vi "Periodic Tasks.vi"(8 "error in":errorcluster) -> ()   [LabVIEW 2020]
doc: "This VI runs in parallel to other tasks. It can contain as many user-defined periodic loops as you need. These can carry out PID or other sorts of timed response."
uses:
  <vilib>/Rock Robotics/WPI/ThirdParty/Phoenix-LabVIEW/Motor Controller/Controls/CTRE_Phoenix_MotorControl_ControlMode.ctl
  swerve_globals.vi
  shooter_globals.vi
  magazine_globals.vi
  climber_globals.vi
  <vilib>/Rock Robotics/WPI/ThirdParty/Phoenix-LabVIEW/Motor Controller/Get/CTRE_Phoenix_MotorController_GetSelectedSensorData.vi
  <vilib>/Rock Robotics/Network Tables/NT Write Number.vi
  <vilib>/Rock Robotics/Network Tables/NT Read Number.vi
  <vilib>/addons/control/pid/pid.llb/PID (DBL).vi
  <vilib>/Rock Robotics/WPI/Utilities/WPI_GetSetVariantRefNum.vi
  TitanLib/Lib/TitanLib.lvlib
  <vilib>/addons/control/pid/NI_PID_pid.lvlib
  <vilib>/Rock Robotics/WPI/ThirdParty/Phoenix-LabVIEW/Motor Controller/Get/CTRE_Phoenix_MotorController_GetVoltage.vi
panel:
  out "Theta":dbl
  in  "Enable Hood":bool
  out "Distance (in)":dbl
  out "Pressure Sensors":T1
  out "Analog  Sensors":cluster{"Analog 0 (V)":dbl, "Analog 1 (V)":dbl}
  in  "Start Compressor":bool
  in  "Stop Compressor":bool
  out "Position (Deg) 2":dbl format="%.2f"
  in  "Zero Turret Encoder 2":bool
  in  "Auto Turret 2":bool
  in  "Min Rotation (deg) 2":dbl=-25.0
  in  "Max Rotation (deg) 2":dbl=20.0
  in  "PID gains":T2={"proportional gain (Kc)"=0.05, "integral time (Ti, min)"=0.0, "derivative time (Td, min)"=0.0} {"derivative time (Td, min)" format="%.3g"; "integral time (Ti, min)" format="%.3e"; "proportional gain (Kc)" format="%.3g"}
  out "tx 2":dbl
  in  "Power Min":dbl
  in  "Climber Up Pos":dbl=-9.82
  in  "Climber Down Pos":dbl=-0.5
  in  "limelight constant":dbl=0.5
  out "Percent Output":dbl(graph)
  out "Setpoint (Deg)":dbl format="%.2f"
  in  "Constants":T3={"Set Constants"=FALSE, "P"=0.05, "I"=0.0, "D"=0.0, "F"=0.0, "I Zone"=0.0, "Cruise Velocity"=500000, "Acceleration"=500000, "Percent Deadband"=0.0}
  out "tx":dbl
  out "Position (Deg)":dbl format="%.2f"
  in  "Zero Turret Encoder":bool
  in  "Min Rotation (deg)":dbl=-45.0
  in  "Max Rotation (deg)":dbl=20.0
  in  "Auto Turret":bool
  out "Loop Time (ms)":u32(graph)
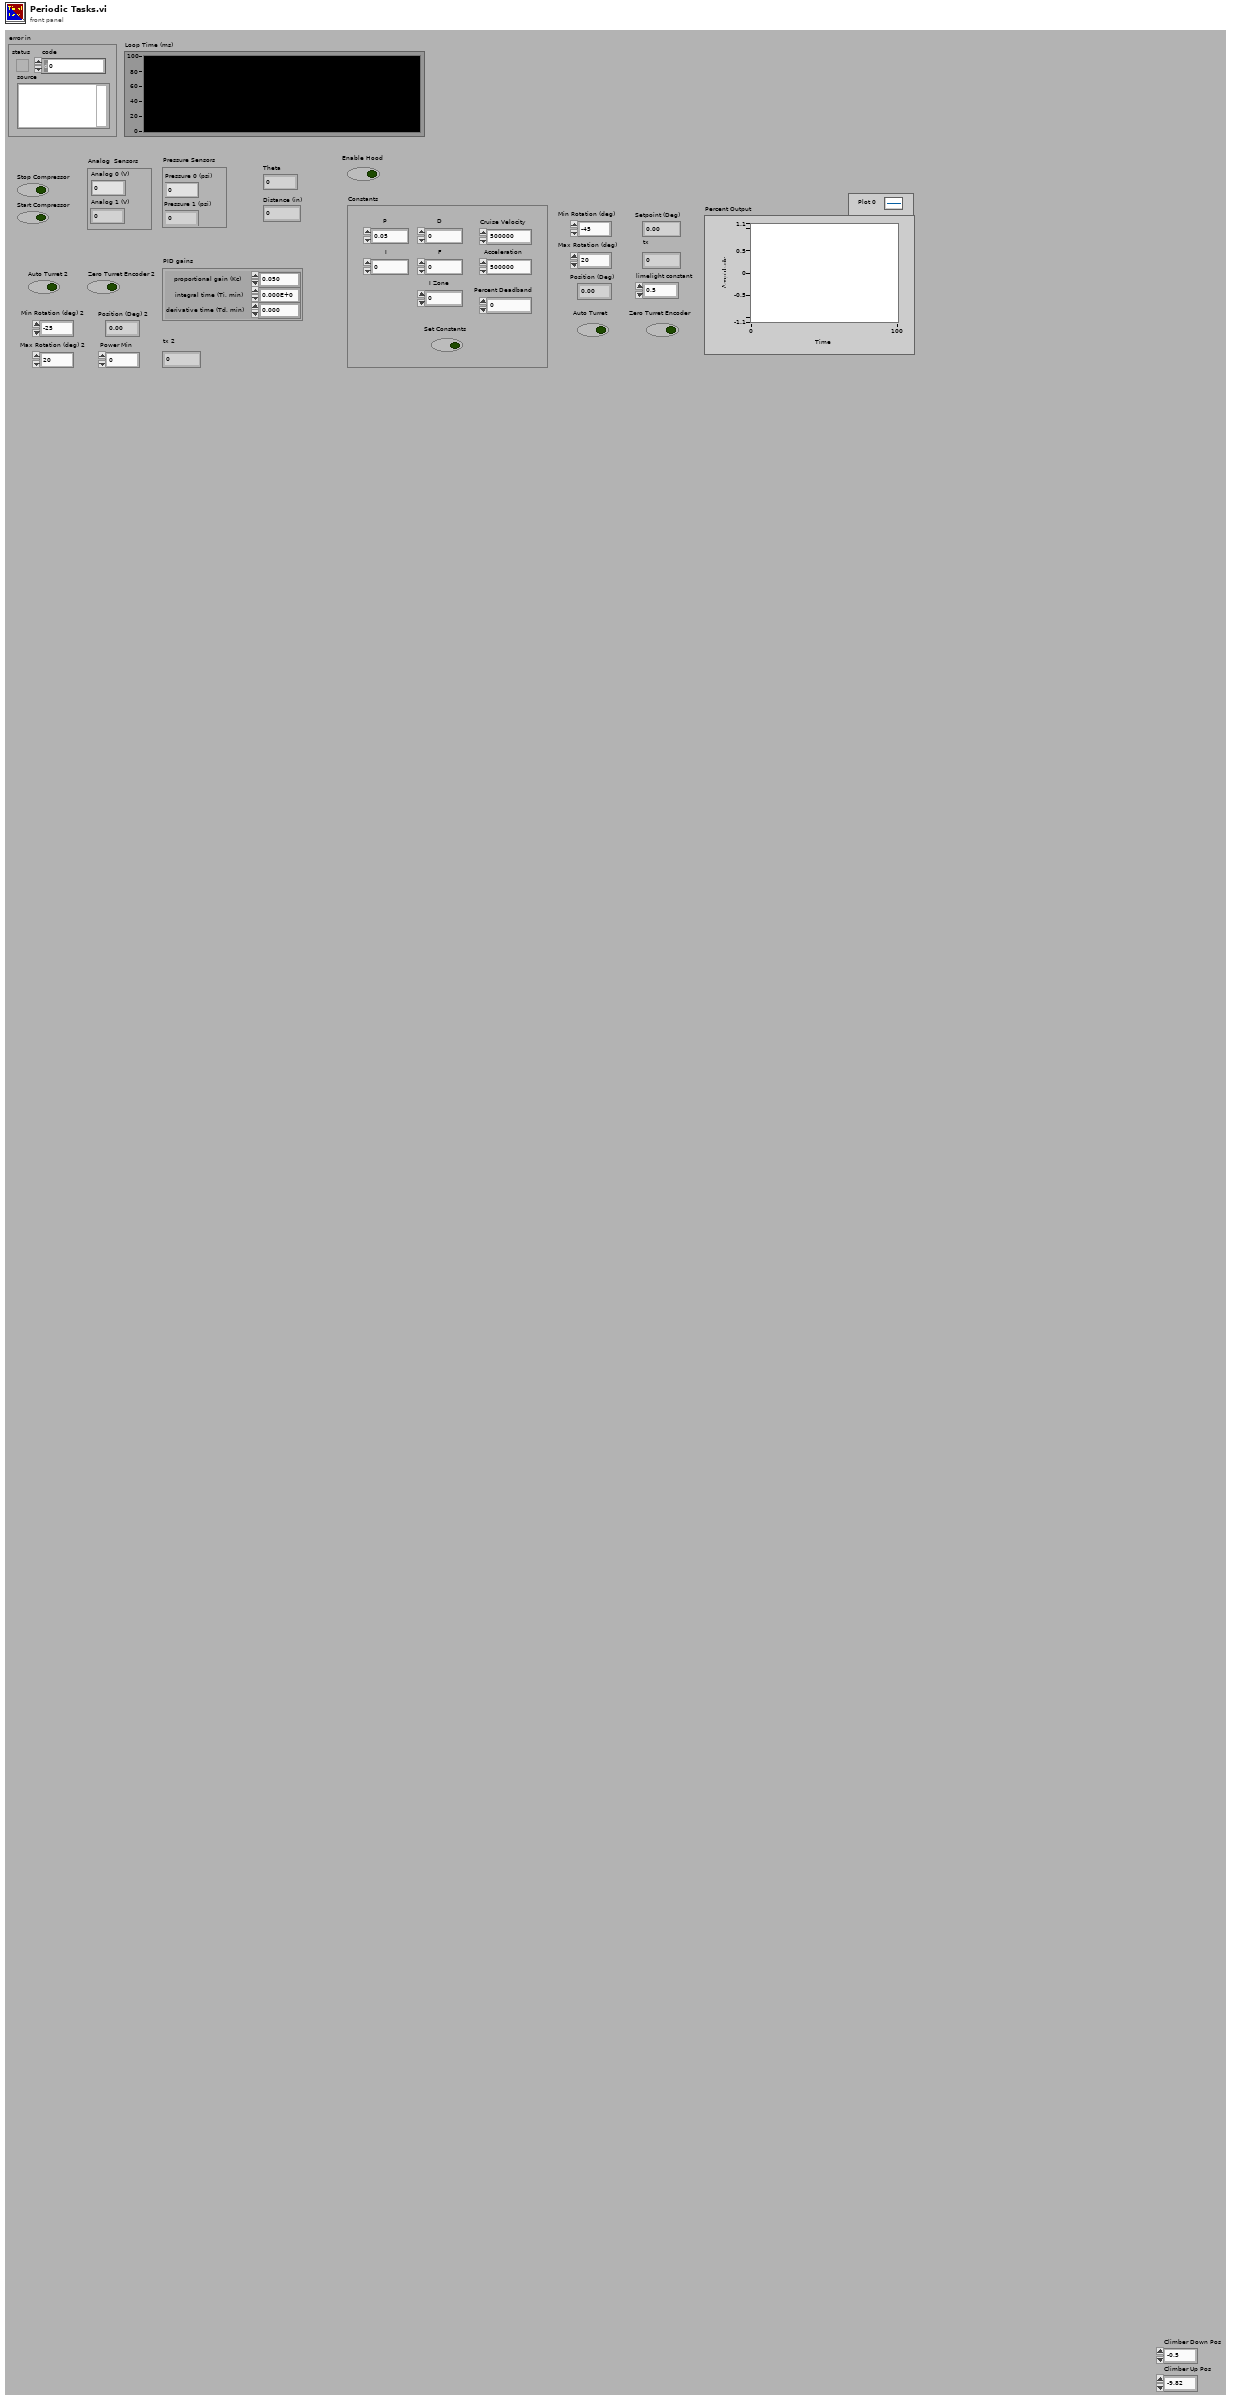
[diagram p1: front panel]
types:
  T1 = cluster{"Pressure 0 (psi)":dbl, "Pressure 1 (psi)":dbl}
  T2 = cluster{"proportional gain (Kc)":dbl, "integral time (Ti, min)":dbl, "derivative time (Td, min)":dbl}
  T3 = cluster{"Set Constants":bool, "P":dbl, "I":dbl, "D":dbl, "F":dbl, "I Zone":dbl, "Cruise Velocity":i32, "Acceleration":i32, "Percent Deadband":dbl}
  T4 = typedef "WPI_CompressorDevRef.ctl" = cluster{"DevStatus":errorcluster, "Pneumatics Control Module":u8}
  T5 = typedef "WPI_MotorControlDeviceRef.ctl" = cluster{"DeviceStatus":errorcluster, "Type":T6, "PWM":cluster{"PWM Channel":T7, "DeadBand":T8}, "CAN":cluster{"Device Number":u8, "SetOutput VI Ref":variant, "GetOutput VI Ref":variant, "Enable VI Ref":variant, "Disable VI Ref":variant, "Data":variant}, "Invert":bool, "DIO PWM":cluster{"PWM \"Enable\" Channel":T7, "DIOChannel":T9, "PWM Rate":dbl}}
  T6 = typedef "WPI_MotorControlType.ctl" = enum16{"PWM", "CAN", "DIO PWM"}
  T7 = typedef "FPGA_DIOPWMChannel.ctl" = enum8{"PWM 0", "PWM 1", "PWM 2", "PWM 3", "PWM 4", "PWM 5", "PWM 6", "PWM 7", "PWM 8", "PWM 9", "PWM MXP 0", "PWM MXP 1", "PWM MXP 2", "PWM MXP 3", "PWM MXP 4", "PWM MXP 5", "PWM MXP 6", "PWM MXP 7", "PWM MXP 8", "PWM MXP 9", "Invalid"}
  T8 = typedef "WPI_PWMDeadband.ctl" = cluster{"Name":string, "maxPositivePwm":i32, "minPositivePwm":i32, "centerPwm":i32, "maxNegativePwm":i32, "minNegativePwm":i32, "angularRange":u16}
  T9 = typedef "FPGA_DIOChannel.ctl" = enum8{"DIO 0", "DIO 1", "DIO 2", "DIO 3", "DIO 4", "DIO 5", "DIO 6", "DIO 7", "DIO 8", "DIO 9", "DIO MXP 0", "DIO MXP 1", "DIO MXP 2", "DIO MXP 3", "DIO MXP 4", "DIO MXP 5", "DIO MXP 6", "DIO MXP 7", "DIO MXP 8", "DIO MXP 9", "DIO MXP 10", "DIO MXP 11", "DIO MXP 12", "DIO MXP 13", "DIO MXP 14", "DIO MXP 15", "SPI Port CS1", "SPI Port CS2", "SPI Port CS3", "SPI Port MISO", "SPI Port MOSI", "Invalid"}
  T10 = typedef "CTRE_Phoenix_MotorControl_ControlMode.ctl" = u16
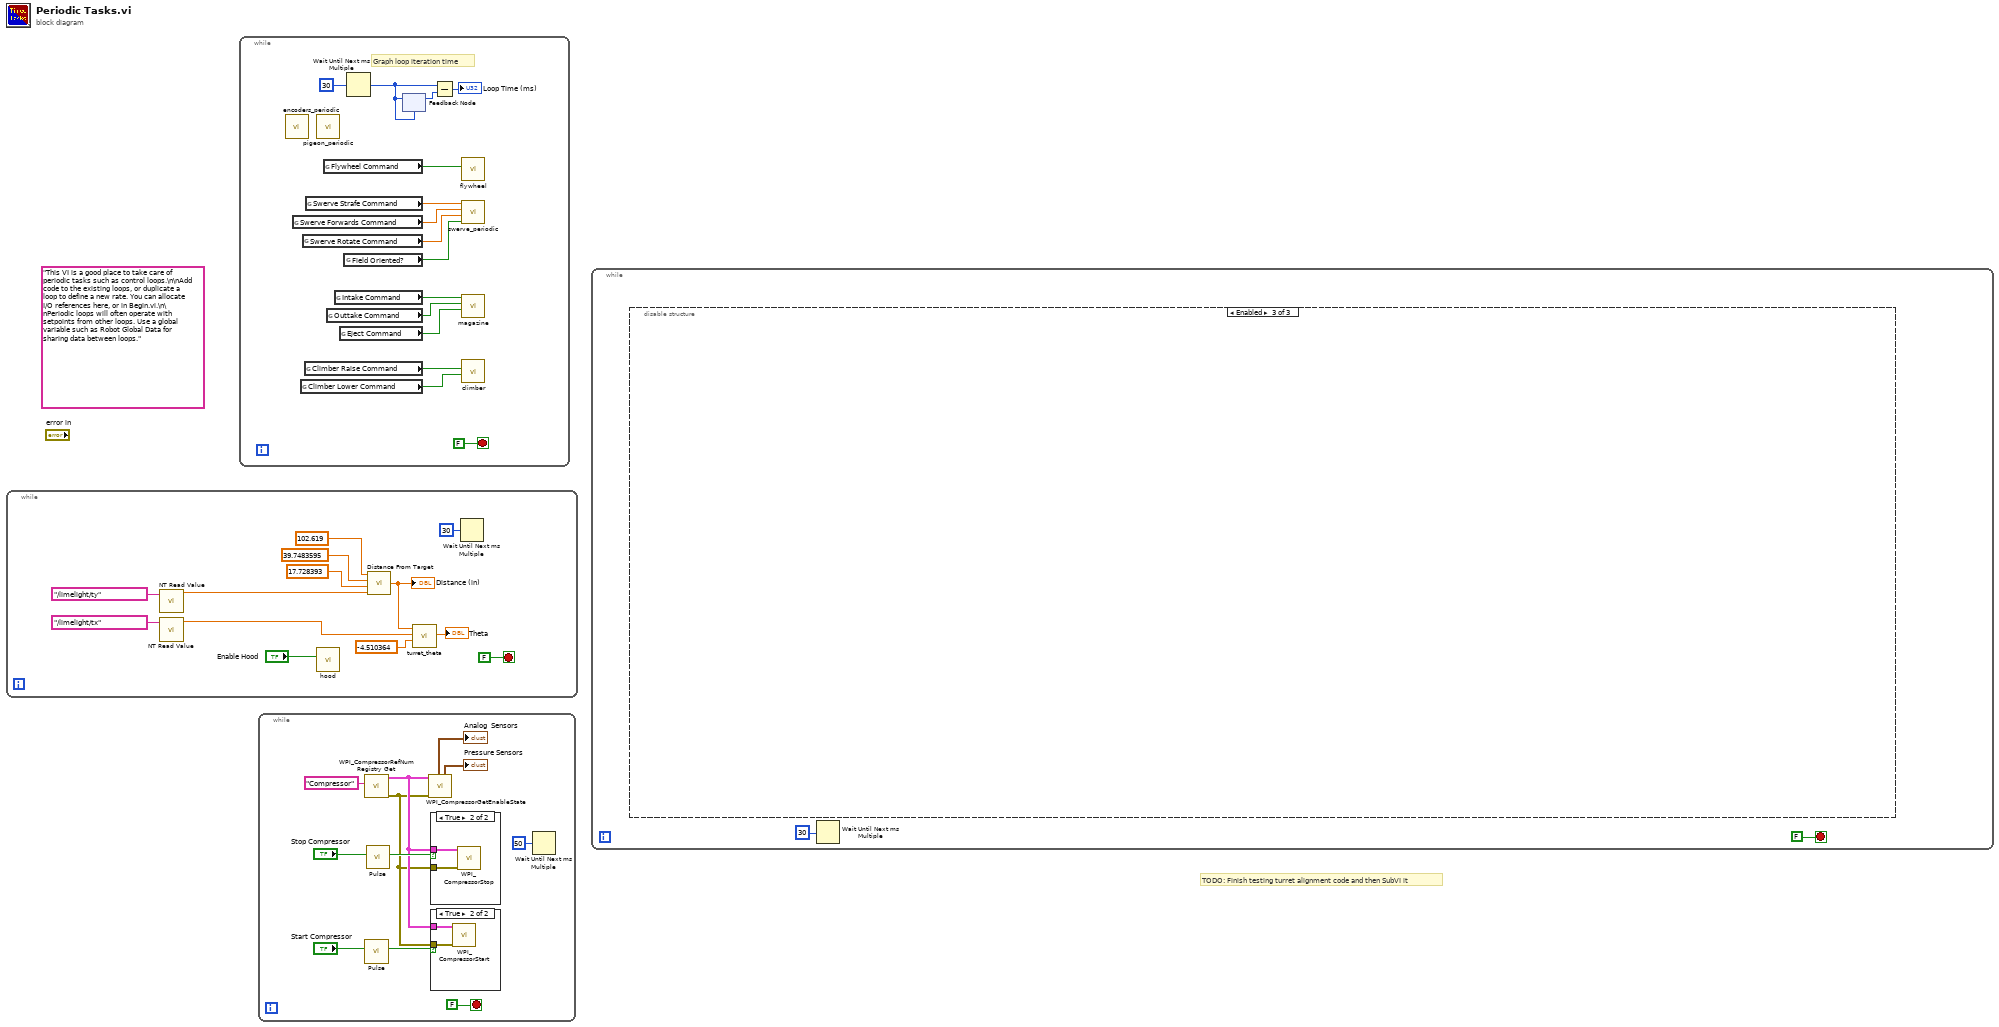
[diagram p0: block diagram]
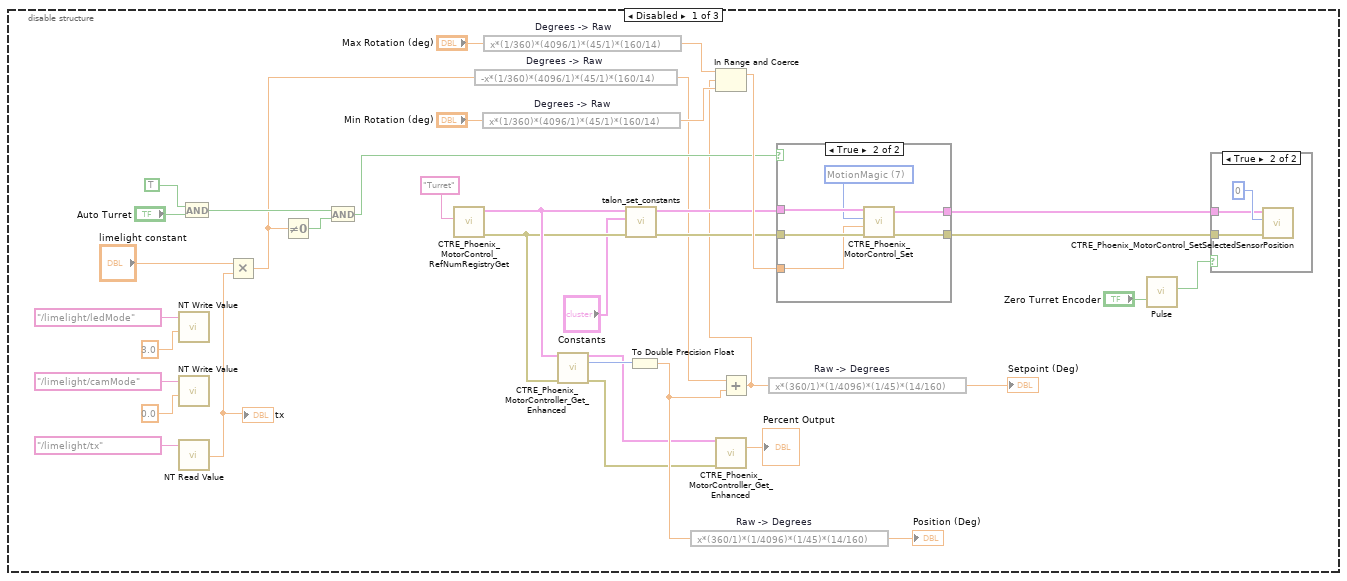
[diagram p4: hidden frame]
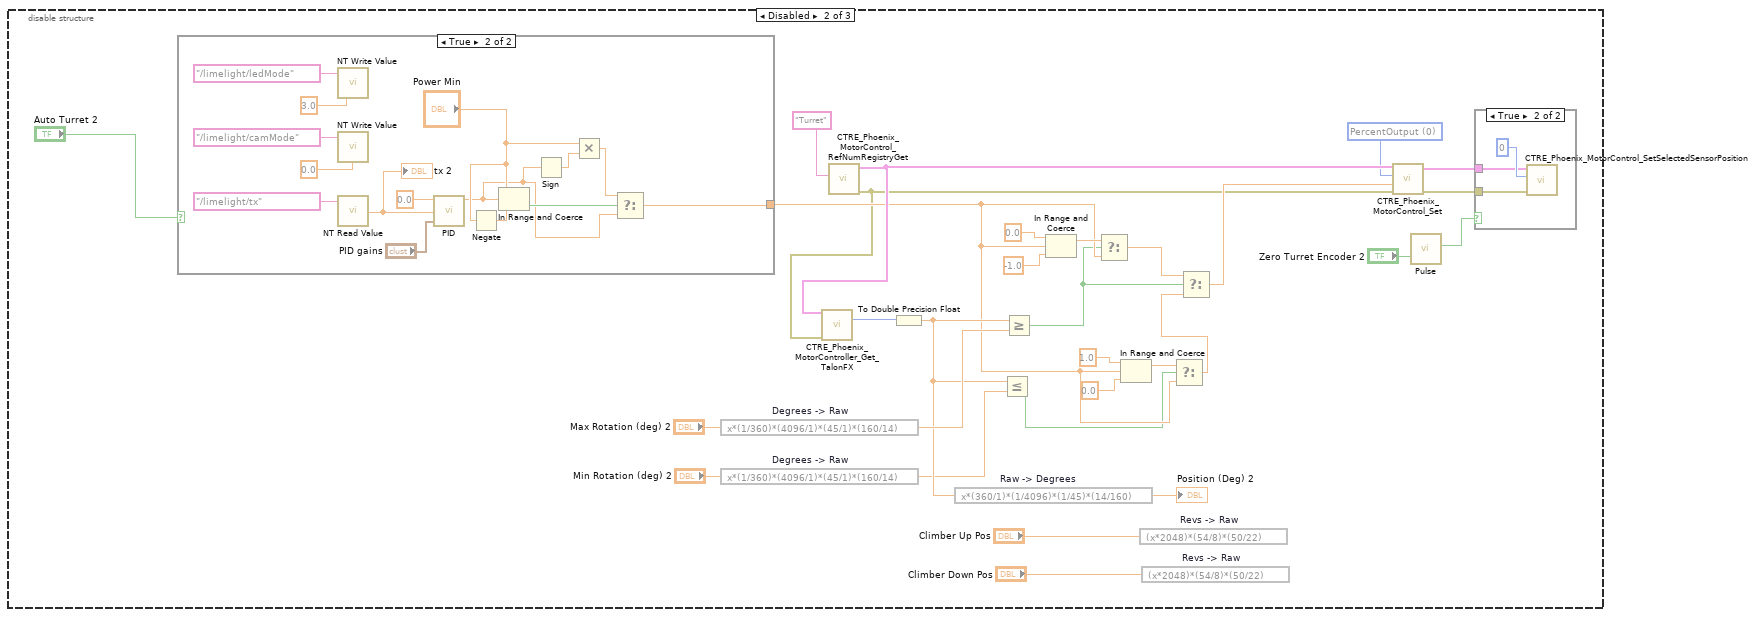
[diagram p7: hidden frame]
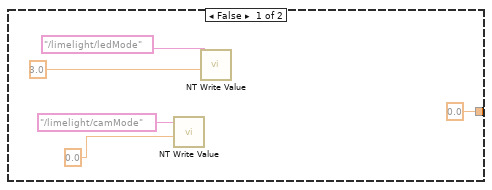
[diagram p9: hidden frame]
diagram:
  (unwired) "This VI is a good place to take care of periodic tasks such as control loops.\n\nAdd code to the existing loops, or duplicate a loop to define a new rate. You can allocate I/O references here, or in Begin.vi.\n\nPeriodic loops will often operate with setpoints from other loops. Use a global variable such as Robot Global Data for sharing data between loops."
  # "TODO: Finish testing turret alignment code and then SubVI it"
  n1 = while {
    stop <- FALSE stop-if-true
    n2 = call-poly <vilib>:"NT Read Value.vi"("Name"="/limelight/ty") -> ("Numeric"=w12:dbl)  [unwired: 9 in, 1 out]
    n3 = call-poly <vilib>:"NT Read Value.vi"("Name"="/limelight/tx") -> ("Numeric"=w4:dbl)  [unwired: 9 in, 1 out]
    n4 = call "hood.vi"("Enable Hood"="Enable Hood") -> ()  [unwired: 11 in]
    n5 = call "Distance From Target.vi"("Target Angle (Deg)"=w12, "Camera Angle (Deg)"=17.728393, "Camera Height (in)"=39.7483595, "Target Height (in)"=102.619) -> ("Distance (in)"=w3:dbl)
    "Distance (in)" <- w3
    n6 = call "turret_theta.vi"("Turret to Limelight Distance (in)"=-4.510364, "Target x (deg)"=w4, "Target Distance (in)"=w3) -> ("Theta"=→"Theta":dbl)  [unwired: 8 in]
    n7 = Wait Until Next ms Multiple(millisecond multiple=u32 30) -> ()  [unwired: 1 out]
  }
  n8 = while {
    stop <- FALSE stop-if-true
    # "Graph loop iteration time"
    n9 = call "encoders_periodic.vi"() -> ()  [unwired: 12 in]
    n10 = global read "swerve_globals.vi" "Swerve Forwards Command"() -> (w22:dbl)
    n11 = global read "climber_globals.vi" "Climber Lower Command"() -> (w14:bool)
    n12 = global read "swerve_globals.vi" "Swerve Rotate Command"() -> (w21:dbl)
    n13 = global read "climber_globals.vi" "Climber Raise Command"() -> (w15:bool)
    n14 = global read "swerve_globals.vi" "Swerve Strafe Command"() -> (w23:dbl)
    n15 = call "pigeon_periodic.vi"() -> ()  [unwired: 12 in]
    n16 = global read "shooter_globals.vi" "Flywheel Command"() -> (w19:bool)
    n17 = global read "magazine_globals.vi" "Outtake Command"() -> (w17:bool)
    n18 = global read "magazine_globals.vi" "Intake Command"() -> (w18:bool)
    n19 = global read "magazine_globals.vi" "Eject Command"() -> (w16:bool)
    n20 = global read "swerve_globals.vi" "Field Oriented?"() -> (w20:bool)
    n21 = Wait Until Next ms Multiple(millisecond multiple=u32 30) -> (millisecond timer value=w25:u32)
    n22 = feedback #1(w25) -> (w28:u32)
    n23 = feedback-in #1(w25) -> ()
    n24 = Subtract(x=w25, y=w28) -> (x-y=→"Loop Time (ms)":u32)
    n25 = call "flywheel.vi"("Flywheel"=w19) -> ()  [unwired: 11 in]
    n26 = call "swerve_periodic.vi"("Field Oriented?"=w20, "Rotate"=w21, "Forwards"=w22, "Strafe"=w23) -> ()  [unwired: 8 in]
    n27 = call "magazine.vi"("Reverse"=w16, "Outtake"=w17, "Intake"=w18) -> ()  [unwired: 9 in]
    n28 = call "climber.vi"("Climber Down"=w14, "Climber Up"=w15) -> ()  [unwired: 10 in]
  }
  n29 = while {
    stop <- FALSE stop-if-true
    n30 = call <vilib>:"WPI_CompressorRefNum Registry Get.vi"("refnum name"="Compressor") -> ("error out"=w33:errorcluster, "CompressorDevRef"=w34:T4)  [unwired: 9 in]
    n31 = call "Pulse.vi"("Input"="Start Compressor") -> ("Output"=w37:bool)  [unwired: 10 in]
    n32 = call "Pulse.vi"("Input"="Stop Compressor") -> ("Output"=w38:bool)  [unwired: 10 in]
    n33 = call <vilib>:"WPI_CompressorGetEnableState.vi"("error in (no error)"=w33, "CompressorDevRef"=w34) -> ("Pressure Sensors"=→"Pressure Sensors":T1, "Analog  Sensors"=→"Analog  Sensors":cluster{"Analog 0 (V)":dbl, "Analog 1 (V)":dbl})  [unwired: 3 in, 5 out]
    n34 = case shown="True" w38 {
      tunnel: w34 -> [_ w43]
      tunnel: w33 -> [_ w42]
      frame False {
      }
      frame True {
        n35 = call <vilib>:"WPI_CompressorStop.vi"("error in (no error)"=w42, "CompressorDevRef"=w43) -> ()  [unwired: 8 in, 2 out]
      }
    }
    n36 = case shown="True" w37 {
      tunnel: w33 -> [_ w41]
      tunnel: w34 -> [_ w40]
      frame False {
      }
      frame True {
        n37 = call <vilib>:"WPI_CompressorStart.vi"("error in (no error)"=w41, "CompressorDevRef"=w40) -> ()  [unwired: 8 in, 2 out]
      }
    }
    n38 = Wait Until Next ms Multiple(millisecond multiple=u32 50) -> ()  [unwired: 1 out]
  }
  n39 = while {
    stop <- FALSE stop-if-true
    n40 = disable-structure shown="Enabled" {
      frame Disabled {
        n41 = call-poly <vilib>:"NT Write Value.vi"("Numeric"=3.0, "Name"="/limelight/ledMode") -> ()  [unwired: 9 in, 1 out]
        n42 = call-poly <vilib>:"NT Write Value.vi"("Numeric"=0.0, "Name"="/limelight/camMode") -> ()  [unwired: 9 in, 1 out]
        n43 = call-poly <vilib>:"NT Read Value.vi"("Name"="/limelight/tx") -> ("Numeric"=w56:dbl)  [unwired: 9 in, 1 out]
        "tx" <- w56
        n44 = And(x=TRUE, y="Auto Turret") -> (x .and. y?=w59:bool)
        n45 = Multiply(x="limelight constant", y=w56) -> (x*y=w47:dbl)
        n46 = Not Equal To 0?(x=w47) -> (x != 0?=w58:bool)
        n47 = And(x=w59, y=w58) -> (x .and. y?=w57:bool)
        n48 = call <vilib>:"CTRE_Phoenix_MotorControl_RefNumRegistryGet.vi"("refnum name"="Turret") -> ("error out"=w63:errorcluster, "PhoenixMotorControlDevRef"=w64:T5)  [unwired: 9 in]
        n49 = expression code="-x*(1/360)*(4096/1)*(45/1)*(160/14)" "Degrees -> Raw"(w47) -> (w55:dbl)
        n50 = expression code="x*(1/360)*(4096/1)*(45/1)*(160/14)" "Degrees -> Raw"("Min Rotation (deg)") -> (w72:dbl)
        n51 = expression code="x*(1/360)*(4096/1)*(45/1)*(160/14)" "Degrees -> Raw"("Max Rotation (deg)") -> (w71:dbl)
        n52 = call-poly <vilib>:"CTRE_Phoenix_MotorController_Get_Enhanced.vi"("PhoenixMotorControlDevRef"=w64, "error in"=w63) -> ("PhoenixMotorControlDevRef"=w51:T5, "Position (Raw Sensor Units)"=w74:i32, "error out"=w50:errorcluster)  [unwired: 10 in, 1 out]
        n53 = call "talon_set_constants.vi"("error in"=w63, "Constants"="Constants", "PhoenixMotorControlDevRef"=w64) -> ("error out"=w61:errorcluster, "PhoenixMotorControlDevRef"=w62:T5)  [unwired: 7 in]
        n54 = To Double Precision Float(number=w74) -> (double precision float=w54:dbl)
        n55 = expression code="x*(360/1)*(1/4096)*(1/45)*(14/160)" "Raw -> Degrees"(w54) -> (→"Position (Deg)":dbl)
        n56 = call-poly <vilib>:"CTRE_Phoenix_MotorController_Get_Enhanced.vi"("PhoenixMotorControlDevRef"=w51, "error in"=w50) -> ("Percent Output"=→"Percent Output":dbl)  [unwired: 9 in, 4 out]
        n57 = Add(x=w55, y=w54) -> (x+y=w53:dbl)
        n58 = In Range and Coerce(upper limit=w71, x=w53, lower limit=w72) -> (coerced(x)=w65:dbl)  [unwired: 1 out]
        n59 = expression code="x*(360/1)*(1/4096)*(1/45)*(14/160)" "Raw -> Degrees"(w53) -> (→"Setpoint (Deg)":dbl)
        n60 = case shown="True" w57 {
          tunnel: w62 -> [w84 w90]
          tunnel: w61 -> [w83 w89]
          tunnel: [w84 w88] -> w78
          tunnel: [w83 w87] -> w77
          tunnel: w65 -> [_ w85]
          frame False {
          }
          frame True {
            w86 = T10 7 items=["PercentOutput"=0, "Position"=1, "Velocity"=2, "Current"=3, "Follower"=5, "MotionProfile"=6, "MotionMagic"=7, "MotionProfileArc"=10, "Disabled"=15] ("Control Mode")
            n61 = call <vilib>:"CTRE_Phoenix_MotorControl_Set.vi"("error in (no error)"=w89, "Output"=w85, "Control Mode"=w86, "PhoenixMotorControlDevRef"=w90) -> ("error out"=w87:errorcluster, "PhoenixMotorControlDevRef"=w88:T5)  [unwired: 6 in]
          }
        }
        n62 = call "Pulse.vi"("Input"="Zero Turret Encoder") -> ("Output"=w76:bool)  [unwired: 10 in]
        n63 = case shown="True" w76 {
          tunnel: w78 -> [_ w92]
          tunnel: w77 -> [_ w91]
          frame False {
          }
          frame True {
            n64 = call <vilib>:"CTRE_Phoenix_MotorControl_SetSelectedSensorPosition.vi"("error in (no error)"=w91, "New Sensor Position"=0, "PhoenixMotorControlDevRef"=w92) -> ()  [unwired: 7 in, 2 out]
          }
        }
      }
      frame Disabled {
        w96 = T10 0 items=["PercentOutput"=0, "Position"=1, "Velocity"=2, "Current"=3, "Follower"=5, "MotionProfile"=6, "MotionMagic"=7, "MotionProfileArc"=10, "Disabled"=15] ("Control Mode")
        n65 = case shown="True" "Auto Turret 2" {
          tunnel: [0.0 ("output") w132] -> w102
          frame False {
            n66 = call-poly <vilib>:"NT Write Value.vi"("Numeric"=0.0, "Name"="/limelight/camMode") -> ()  [unwired: 9 in, 1 out]
            n67 = call-poly <vilib>:"NT Write Value.vi"("Numeric"=3.0, "Name"="/limelight/ledMode") -> ()  [unwired: 9 in, 1 out]
          }
          frame True {
            n68 = call-poly <vilib>:"NT Write Value.vi"("Numeric"=3.0, "Name"="/limelight/ledMode") -> ()  [unwired: 9 in, 1 out]
            n69 = call-poly <vilib>:"NT Write Value.vi"("Numeric"=0.0, "Name"="/limelight/camMode") -> ()  [unwired: 9 in, 1 out]
            n70 = call-poly <vilib>:"NT Read Value.vi"("Name"="/limelight/tx") -> ("Numeric"=w137:dbl)  [unwired: 9 in, 1 out]
            "tx 2" <- w137
            n71 = call-poly <vilib>:"PID.vi"("PID gains"="PID gains", "process variable"=w137, "setpoint"=0.0) -> ("output"=w133:dbl)  [unwired: 7 in, 1 out]
            n72 = Negate(x="Power Min") -> (-x=w139:dbl)
            n73 = In Range and Coerce(upper limit="Power Min", x=w133, lower limit=w139) -> (In Range?=w138:bool)  [unwired: 1 out]
            n74 = Sign(1:w133) -> (0:w136:dbl)
            n75 = Multiply(x="Power Min", y=w136) -> (x*y=w134:dbl)
            n76 = Select(t=w134, s=w138, f=w133) -> (s? t:f=w132:dbl)
          }
        }
        n77 = expression code="x*(1/360)*(4096/1)*(45/1)*(160/14)" "Degrees -> Raw"("Max Rotation (deg) 2") -> (w119:dbl)
        n78 = expression code="x*(1/360)*(4096/1)*(45/1)*(160/14)" "Degrees -> Raw"("Min Rotation (deg) 2") -> (w109:dbl)
        n79 = call <vilib>:"CTRE_Phoenix_MotorControl_RefNumRegistryGet.vi"("refnum name"="Turret") -> ("error out"=w94:errorcluster, "PhoenixMotorControlDevRef"=w120:T5)  [unwired: 9 in]
        n80 = call-poly <vilib>:"CTRE_Phoenix_MotorController_Get_TalonFX.vi"("PhoenixMotorControlDevRef"=w120, "error in"=w94) -> ("Position (Raw Sensor Units)"=w112:i32)  [unwired: 10 in, 3 out]
        n81 = To Double Precision Float(number=w112) -> (double precision float=w111:dbl)
        n82 = expression code="x*(360/1)*(1/4096)*(1/45)*(14/160)" "Raw -> Degrees"(w111) -> (→"Position (Deg) 2":dbl)
        n83 = Less Or Equal?(x=w111, y=w109) -> (x <= y?=w101:bool)
        n84 = Greater Or Equal?(x=w111, y=w119) -> (x >= y?=w100:bool)
        n85 = In Range and Coerce(upper limit=0.0, x=w102, lower limit=-1.0) -> (coerced(x)=w106:dbl)  [unwired: 1 out]
        n86 = Select(t=w106, s=w100, f=w102) -> (s? t:f=w99:dbl)
        n87 = In Range and Coerce(upper limit=1.0, x=w102, lower limit=0.0) -> (coerced(x)=w105:dbl)  [unwired: 1 out]
        n88 = expression code="(x*2048)*(54/8)*(50/22)" "Revs -> Raw"("Climber Up Pos") -> ()  [unwired: 1 out]
        n89 = expression code="(x*2048)*(54/8)*(50/22)" "Revs -> Raw"("Climber Down Pos") -> ()  [unwired: 1 out]
        n90 = Select(t=w105, s=w101, f=w102) -> (s? t:f=w98:dbl)
        n91 = Select(t=w99, s=w100, f=w98) -> (s? t:f=w97:dbl)
        n92 = call <vilib>:"CTRE_Phoenix_MotorControl_Set.vi"("error in (no error)"=w94, "Output"=w97, "Control Mode"=w96, "PhoenixMotorControlDevRef"=w120) -> ("error out"=w115:errorcluster, "PhoenixMotorControlDevRef"=w116:T5)  [unwired: 6 in]
        n93 = call "Pulse.vi"("Input"="Zero Turret Encoder 2") -> ("Output"=w114:bool)  [unwired: 10 in]
        n94 = case shown="True" w114 {
          tunnel: w116 -> [_ w125]
          tunnel: w115 -> [_ w124]
          frame False {
          }
          frame True {
            n95 = call <vilib>:"CTRE_Phoenix_MotorControl_SetSelectedSensorPosition.vi"("error in (no error)"=w124, "New Sensor Position"=0, "PhoenixMotorControlDevRef"=w125) -> ()  [unwired: 7 in, 2 out]
          }
        }
      }
      frame Enabled {
      }
    }
    n96 = Wait Until Next ms Multiple(millisecond multiple=u32 30) -> ()  [unwired: 1 out]
  }
